vi "tdms test.vi"(11 "logrotate_options":T1={"max file size (bytes)"=10000, "rotate count"=5, "max age (days)"=3.0, "No archive dir"=FALSE, "Archive dir"=path ""}) -> (0 "error out":errorcluster, 3 "found?":bool)   [LabVIEW 2013, in "tdms logger tests.lvlib"]
uses:
  tdms logger tests.lvlib
  configuration/TDMS datalogger configuration.lvclass
  execution/TDMS datalogger runtime.lvclass
  <vilib>/NI/Tag Bus Module Framework/channel/TBM channel.lvclass
  <vilib>/NI/Tag Bus Module Framework/channel/channel classification.ctl
  <vilib>/NI/Tag Bus/tag/Data Type.ctl
  <vilib>/NI/Tag Bus/tag/tag descriptor.lvclass
  <vilib>/NI/Tag Bus/table/data table.lvlib
  <vilib>/platform/TimedLoop/XDataNode/XDataNode.xnode
  <vilib>/Platform/TimedLoop/XDataNode/nitl_modes.ctl
  <vilib>/Platform/TimedLoop/XDataNode/XDNodeRunTimeDep.lvlib
  <vilib>/Platform/TimedLoop/XDataNode/wakeup.ctl
  <vilib>/Platform/TimedLoop/XDataNode/timing_clust.ctl
  <vilib>/NI/Tag Bus/table/data polymorphs/write one/write Boolean.vi
  <vilib>/Utility/RT CPU pool selections.ctl
  <vilib>/NI/Configuration Framework/serializable configuration/NISE_CEF_serializable configuration.lvclass
  <vilib>/NI/LogRotate/options.ctl
  <vilib>/NI/LogRotate/LogRotate.lvclass
panel:
  in  "iterations":i32=1000
  in  "scans per write":i32=20
  in  "queue size":i32=20
  out "max":dbl
  out "min":dbl
  in  "enable state":bool=TRUE
  in  "stop":bool
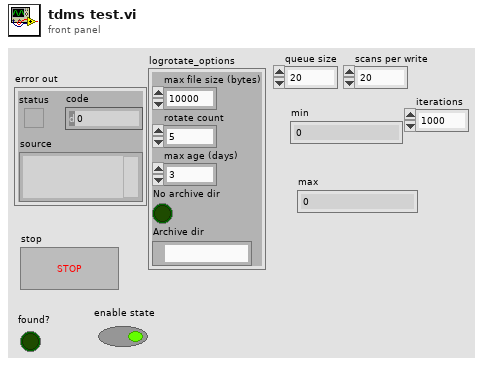
[diagram p1: front panel]
types:
  T1 = typedef "LogRotate.lvclass/options.ctl" = cluster{"max file size (bytes)":i64, "rotate count":u32, "max age (days)":dbl, "No archive dir":bool, "Archive dir":path}
  T2 = typedef "tag bus.lvlib/tag descriptor.lvclass/Data Type.ctl" = enum16{"Double", "Single", "I64", "I32", "I16", "I8", "U64", "U32", "U16", "U8", "Boolean", "String", "Array of Double", "Array of Single", "Array of I64", "Array of I32", "Array of I16", "Array of I8", "Array of U64", "Array of U32", "Array of U16", "Array of U8", "Array of Boolean", "Array of String"}
  T3 = typedef "TBM channel.lvclass/channel classification.ctl" = enum16{"input data", "output data", "processing parameter", "processing result"}
  T4 = typedef "NI_Real-Time Target Support.lvlib/RT CPU pool selections.ctl" = enum16{"System & Timed Structures", "System", "Timed Structures", "Reserved"}
  T5 = typedef "TBM channel.lvclass/data tables.ctl" = cluster{"input data":T6, "processing parameter":T6, "processing result":T6, "output data":T6}
  T6 = typedef "tag bus.lvlib/dictionary table pair.ctl" = cluster{"data dictionary":refnum<class "data dictionary.lvclass">, "data table":T7}
  T7 = typedef "tag bus.lvlib/data table.lvlib/data table.ctl" = cluster{"Double":dbl[], "Single":sgl[], "I64":i64[], "I32":i32[], "I16":i16[], "I8":i8[], "U64":u64[], "U32":u32[], "U16":u16[], "U8":u8[], "Boolean":bool[], "String":string[], "Array of Double":cluster{"DBL Array":dbl[]}[], "Array of Single":cluster{"SGL Array":sgl[]}[], "Array of I64":cluster{"I64 Array":i64[]}[], "Array of I32":cluster{"I32 Array":i32[]}[], "Array of I16":cluster{"I16 Array":i16[]}[], "Array of I8":cluster{"I8 Array":i8[]}[], "Array of U64":cluster{"U64 Array":u64[]}[], "Array of U32":cluster{"U32 Array":u32[]}[], "Array of U16":cluster{"U16 Array":u16[]}[], "Array of U8":cluster{"U8 Array":u8[]}[], "Array of Boolean":cluster{"Boolean Array":bool[]}[], "Array of String":cluster{"String Array":string[]}[]}
  T8 = typedef "XDNodeRunTimeDep.lvlib/timing_clust.ctl" = cluster{"Expected End [f-1]":u64, "Actual End [f-1]":u64, "Finished Late? [f-1]":bool, "Expected End [i-1]":u64, "Actual End [i-1]":u64, "Finished Late? [i-1]":bool, "Expected Start [i]":u64, "Actual Start [i]":u64, "Expected Start [f]":u64, "Actual Start [f]":u64, "Source Name":string, "Structure Name":string, "Period":i64, "Deadline":i64, "Offset":i64, "Start":i64, "Priority":i32, "Timeout":i32, "Mode":T9, "Wakeup Reason":T10, "Error":errorcluster, "Source Type":string, "Secondary Source Type":string, "Global End Time":u64, "Global Start Time":u64, "Frame Duration":u64, "Iteration Duration":u64, "Assigned CPU":i32, "I/O Scan Engine Mode":u32}
  T9 = typedef "XDNodeRunTimeDep.lvlib/nitl_modes.ctl" = enum32{"No Change", "Process missed periods, maintain original phase", "Discard missed periods, maintain original phase", "Process missed periods, ignore original phase", "Discard missed periods, ignore original phase"}
  T10 = typedef "XDNodeRunTimeDep.lvlib/wakeup.ctl" = enum32{"Normal", "Aborted", "Asynchronous wakeup", "Timing source error", "Timed loop error", "Timeout"}
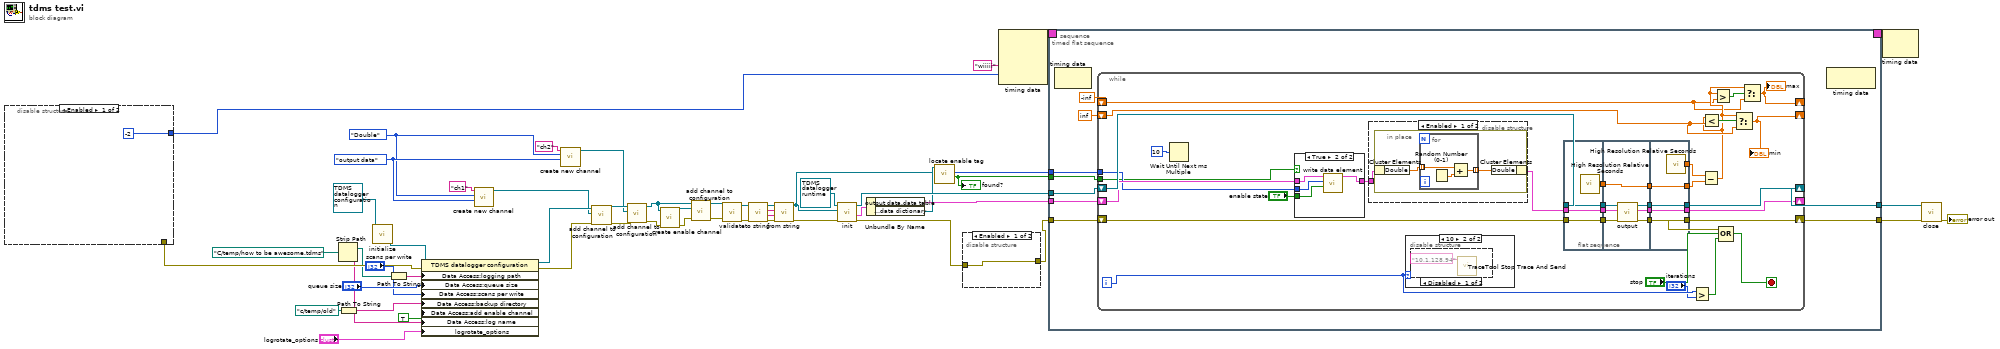
[diagram p0: block diagram]
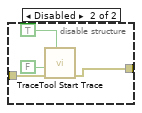
[diagram p2: hidden frame]
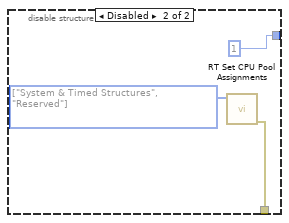
[diagram p3: hidden frame]
diagram:
  w37 = Data_Type."Double" ("data type")
  w38 = channel_classification."output data" ("channel classification")
  n1 = disable-structure shown="Enabled" {
    disable-tunnel: [_ w56] -> w25
    disable-tunnel: [-2 ("Processor") 1 ("Processor")] -> w24
    frame Enabled {
    }
    frame Disabled {
      w57 = T4[] [enum."System & Timed Structures", enum."Reserved"] items=["System & Timed Structures", "System", "Timed Structures", "Reserved"] ("CPU pools")
      n2 = call <vilib>:"RT Set CPU Pool Assignments.vi"("CPU pools"=w57) -> ("error out"=w56:errorcluster)  [unwired: 7 in, 3 out]
    }
  }
  n3 = Strip Path(path=path "C:/temp/how to be awesome.tdms" ("output file path")) -> (stripped path=w5:path, name=w3:string)
  n4 = Path To String(path=path "c:/temp/old" ("output file path")) -> (string=w2:string)
  n5 = call <vilib>:"initialize.vi"("configuration in"=refnum<class "TDMS datalogger configuration.lvclass"> refnum ("TDMS datalogger configuration")) -> ("configuration out"=w7:refnum<class "TDMS datalogger configuration.lvclass">)  [unwired: 8 in, 2 out]
  n6 = Path To String(path=w5) -> (string=w4:string)
  n7 = property class="TDMS datalogger configuration"(reference=w7, error in=w25, "Data Access:logging path"=w4, "Data Access:queue size"="queue size", "Data Access:scans per write"="scans per write", "Data Access:backup directory"=w2, "Data Access:add enable channel"=TRUE ("add enable channel"), "Data Access:log name"=w3, "logrotate_options"="logrotate_options") -> (reference out=w17:refnum<class "TDMS datalogger configuration.lvclass">, error out=w16:errorcluster)
  n8 = call <vilib>:"create new channel.vi"("channel classification"=w38, "data type"=w37, "channel name"="ch1") -> ("channel"=w15:refnum<class "TBM channel.lvclass">)  [unwired: 8 in]
  n9 = call <vilib>:"create new channel.vi"("channel classification"=w38, "data type"=w37, "channel name"="ch2") -> ("channel"=w13:refnum<class "TBM channel.lvclass">)  [unwired: 8 in]
  n10 = call "add channel to configuration.vi"("error in"=w16, "TBM channel in"=w15, "TDMS datalogger configuration in"=w17) -> ("error out"=w14:errorcluster, "TDMS datalogger configuration out"=w18:refnum<class "TDMS datalogger configuration.lvclass">)  [unwired: 7 in]
  n11 = call "add channel to configuration.vi"("error in"=w14, "TBM channel in"=w13, "TDMS datalogger configuration in"=w18) -> ("error out"=w10:errorcluster, "TDMS datalogger configuration out"=w9:refnum<class "TDMS datalogger configuration.lvclass">)  [unwired: 7 in]
  n12 = call "create enable channel.vi"("error in"=w10, "TDMS datalogger configuration"=w9) -> ("error out"=w11:errorcluster, "enable channel"=w12:refnum<class "TBM channel.lvclass">)  [unwired: 7 in, 1 out]
  n13 = call "add channel to configuration.vi"("error in"=w11, "TBM channel in"=w12, "TDMS datalogger configuration in"=w9) -> ("error out"=w20:errorcluster, "TDMS datalogger configuration out"=w19:refnum<class "TDMS datalogger configuration.lvclass">)  [unwired: 7 in]
  n14 = call-dynamic "validate.vi"("error in"=w20, "TDMS datalogger configuration in"=w19) -> ("error out"=w53:errorcluster, "TDMS datalogger configuration out"=w52:refnum<class "TDMS datalogger configuration.lvclass">)  [unwired: 8 in]
  n15 = call-dynamic "to string.vi"("error in"=w53, "TDMS datalogger configuration in"=w52) -> ("error out"=w50:errorcluster, "data"=w49:string, "version"=w48:string, "TDMS datalogger configuration out"=w51:refnum<class "TDMS datalogger configuration.lvclass">)  [unwired: 6 in]
  n16 = call-dynamic "from string.vi"("error in"=w50, "data"=w49, "version"=w48, "TDMS datalogger configuration in"=w51) -> ("error out"=w47:errorcluster, "TDMS datalogger configuration out"=w8:refnum<class "TDMS datalogger configuration.lvclass">)  [unwired: 6 in]
  n17 = call-dynamic "init.vi"("error in"=w47, "TBM module configuration in"=w8, "TDMS datalogger runtime in"=refnum<class "TDMS datalogger runtime.lvclass"> refnum ("TDMS datalogger runtime")) -> ("error out"=w23:errorcluster, "data allocations"=w39:T5, "TDMS datalogger runtime out"=w46:refnum<class "TDMS datalogger runtime.lvclass">)  [unwired: 5 in, 1 out]
  n18 = Unbundle By Name(w39) -> ("output data.data table"=w45:T7, "output data.data dictionary"=w30:refnum<class "data dictionary.lvclass">)
  n19 = call "locate enable tag.vi"("TDMS datalogger configuration"=w8, "data dictionary in"=w30) -> ("found?"=w28:bool, "index"=w29:i32)  [unwired: 7 in, 1 out]
  "found?" <- w28
  n20 = disable-structure shown="Enabled" {
    disable-tunnel: [w58 w61] -> w22
    disable-tunnel: w23 -> [w58 w62]
    frame Enabled {
    }
    frame Disabled {
      n21 = call <vilib>:"TraceTool Start Trace.vi"("Detailed Tracing? (F)"=TRUE, "error in (no error)"=w62, "VI Tracing? (T)"=FALSE) -> ("error out"=w61:errorcluster)  [unwired: 7 in, 1 out]
    }
  }
  n22 = node-c288("wiiiii" ("Structure Name"), w24) -> (w27:T8)  [unwired: 2 in]
  n23 = timed-sequence {
    timing: w27 -> [_]
    timing-out: [_] -> w26
    tunnel: w46 -> [w69]
    tunnel: w22 -> [w68]
    tunnel: w45 -> [w67]
    tunnel: [w66] -> w44
    tunnel: [w65] -> w43
    tunnel: w29 -> [w64]
    tunnel: w28 -> [w63]
    n24 = timed-flat-sequence {
      tunnel: w69 -> [w78]
      tunnel: w68 -> [w77]
      tunnel: w67 -> [w76]
      tunnel: [w75] -> w66
      tunnel: [w74] -> w65
      tunnel: w64 -> [w73]
      tunnel: w63 -> [w72]
      n25 = node-c288() -> ()  [unwired: 1 in, 1 out]
      n26 = while {
        shift-right: [w100] -> w74
        shift-left: w77 -> [w111]
        shift-right: [w110] -> w75
        shift-left: w78 -> [w112]
        shift-right: [w108] -> _
        shift-left: w76 -> [w105]
        tunnel: w73 -> [w103]
        tunnel: w72 -> [w102]
        shift-right: [w83] -> _
        shift-left: -inf -> [w85]
        shift-right: [w84] -> _
        shift-left: inf -> [w87]
        i -> [w81]
        stop <- w101 stop-if-true
        n27 = Wait Until Next ms Multiple(millisecond multiple=u32 10) -> ()  [unwired: 1 out]
        n28 = case shown="True" w102 {
          tunnel: w105 -> [w113 w117]
          tunnel: [w113 w116] -> w104
          tunnel: w103 -> [_ w115]
          tunnel: "enable state" -> [_ w114]
          frame False {
          }
          frame True {
            n29 = call-poly <vilib>:"write data element.vi"("value"=w114, "index"=w115, "data table in"=w117) -> ("data table out"=w116:T7)  [unwired: 8 in]
          }
        }
        n30 = disable-structure shown="Enabled" {
          disable-tunnel: [w136 w142] -> w109
          disable-tunnel: w104 -> [w135 w142]
          frame Enabled {
            n31 = in-place {
              n32 = in-place-cluster #1(w135) -> ("Double"=w138:dbl[])
              n33 = for {
                tunnel: w138 -> [w141] mode=indexing
                tunnel: [w140] -> w137 mode=indexing
                n34 = Random Number (0-1)() -> (number: 0 to 1=w139:dbl)
                n35 = Add(x=w141, y=w139) -> (x+y=w140:dbl)
              }
              n36 = in-place-cluster #1("Double"=w137) -> (w136:T7)
            }
          }
          frame Disabled {
          }
        }
        n37 = case shown="10" w81 {
          frame 0, Default {
          }
          frame 10 {
            n38 = disable-structure shown="Disabled" {
              frame Disabled {
                n39 = call <vilib>:"TraceTool Stop Trace And Send.vi"("Trace Host Network Address"="10.1.128.94") -> ()  [unwired: 10 in, 1 out]
              }
              frame Enabled {
              }
            }
          }
        }
        n40 = flat-sequence {
          tunnel: w109 -> [w120]
          tunnel: w111 -> [w121]
          tunnel: w112 -> [w122]
          tunnel: [w122] -> w96
          tunnel: [w121] -> w95
          tunnel: [w120] -> w94
          tunnel: [w119] -> w92
          tunnel: [w127] -> w99
          tunnel: [w125] -> w98
          tunnel: [w124] -> w97
          tunnel: w96 -> [w129]
          tunnel: w95 -> [w128]
          tunnel: w94 -> [w126]
          tunnel: [w123] -> w93
          tunnel: w92 -> [w123]
          tunnel: [w132] -> w100
          tunnel: [w133] -> w108
          tunnel: [w134] -> w110
          tunnel: w99 -> [w134]
          tunnel: w98 -> [w133]
          tunnel: w97 -> [w132]
          tunnel: [w131] -> w91
          tunnel: w93 -> [w131]
          tunnel: [w130] -> w90
          frame #0 {
            n41 = call <vilib>:"High Resolution Relative Seconds.vi"() -> ("relative seconds"=w119:dbl)
          }
          frame #1 {
            n42 = call-dynamic "output.vi"("error in"=w128, "data table in"=w126, "TDMS datalogger runtime in"=w129) -> ("error out"=w124:errorcluster, "data table out"=w125:T7, "TDMS datalogger runtime out"=w127:refnum<class "TDMS datalogger runtime.lvclass">)  [unwired: 6 in]
          }
          frame #2 {
            n43 = call <vilib>:"High Resolution Relative Seconds.vi"() -> ("relative seconds"=w130:dbl)
          }
        }
        n44 = Greater?(x=w81, y="iterations") -> (0:w79:bool)
        n45 = Subtract(x=w90, y=w91) -> (x-y=w86:dbl)
        n46 = Less?(x=w86, y=w87) -> (x < y?=w88:bool)
        n47 = Greater?(x=w86, y=w85) -> (0:w89:bool)
        n48 = Compound Arithmetic op=OR(w100, "stop", w79) -> (w101:bool)
        n49 = Select(t=w86, s=w88, f=w87) -> (s? t:f=w84:dbl)
        "min" <- w84
        n50 = Select(t=w86, s=w89, f=w85) -> (s? t:f=w83:dbl)
        "max" <- w83
      }
      n51 = node-c288() -> ()  [unwired: 1 in, 1 out]
    }
  }
  n52 = node-c288(w26) -> ()  [unwired: 1 out]
  n53 = call-dynamic "close.vi"("error in"=w43, "TDMS datalogger runtime in"=w44) -> ("error out"=→"error out":errorcluster)  [unwired: 9 in]
